vi "tls_security.vi"   [LabVIEW 2023]
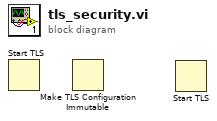
[diagram p0: block diagram]
diagram:
  n1 = Start TLS() -> ()  [unwired: 6 in, 3 out]
  n2 = Make TLS Configuration Immutable() -> ()  [unwired: 2 in, 2 out]
  n3 = Start TLS() -> ()  [unwired: 6 in, 3 out]
